vi "Actor-Run.vi"(8 "error in":errorcluster, 9 "Actor-Event-Registrations":T2, 10 "Actor-Events":T1, 11 "Actor in":refnum<class "Actor.lvclass">) -> (0 "error out":errorcluster, 3 "Actor out":refnum<class "Actor.lvclass">)   [LabVIEW 2018, in "Actor.lvlib" / "Actor.lvclass"]
uses:
  Actor.lvclass
  Event-Registrations.ctl
  Stop.ctl
  Events.ctl
  Launched.ctl
  Actor-Interface.lvclass
types:
  T1 = typedef "Actor.lvlib/Actor-Interface.lvclass/Events.ctl" = cluster{"Stop":refnum<user-event>, "Launched":refnum<user-event>}
  T2 = typedef "Actor.lvlib/Actor-Interface.lvclass/Event-Registrations.ctl" = cluster{"Stop":refnum<event-registration>}
  T3 = typedef "Actor.lvlib/Actor-Interface.lvclass/Launched.ctl" = cluster{"Actor":refnum<class "Actor.lvclass">}
  T4 = typedef "Actor.lvlib/Actor-Interface.lvclass/Stop.ctl" = enum16{"Normal", "Emergency"}
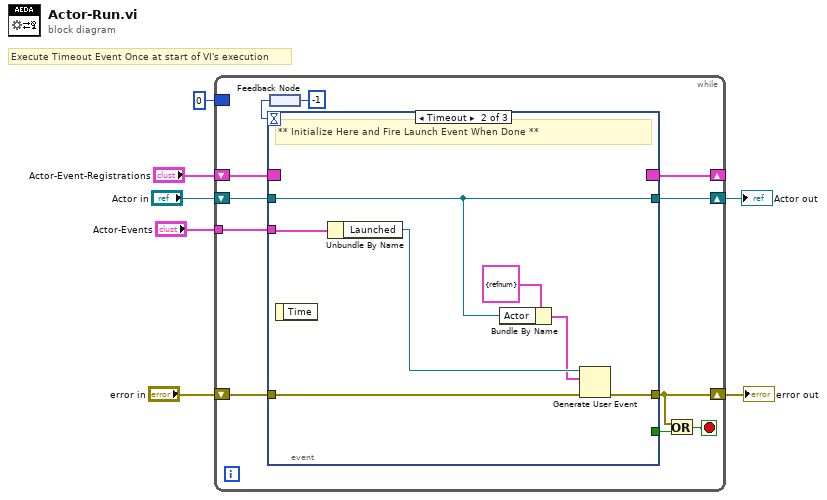
[diagram p0: block diagram]
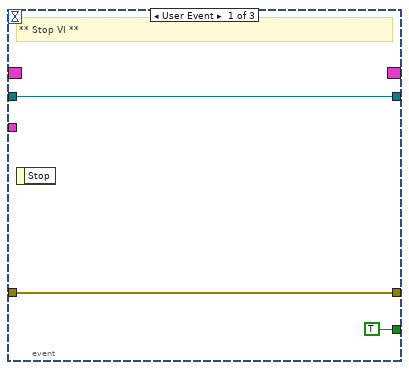
[diagram p2: hidden frame]
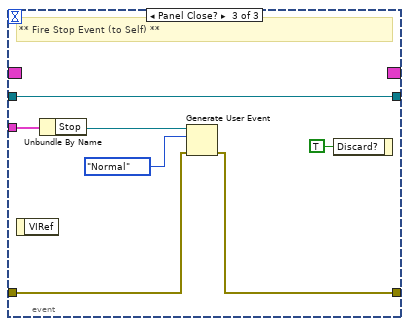
[diagram p3: hidden frame]
diagram:
  # "Execute Timeout Event Once at start of VI's execution"
  n1 = while {
    shift-right: [w13] -> w3
    shift-left: "Actor in" -> [w18]
    shift-right: [w12] -> w2
    shift-left: "error in" -> [w16]
    tunnel: "Actor-Events" -> [w15]
    shift-right: [w14] -> _
    shift-left: "Actor-Event-Registrations" -> [w17]
    border: 0 -> [_]
    stop <- w10 stop-if-true
    n2 = feedback-in #1(-1) -> ()
    n3 = feedback #1() -> (w8:i32)
    n4 = event shown="[1] Timeout" {
      selector: w17 -> [_ _ _]
      dyn-events: [_ _ _] -> w14
      timeout: w8 -> [_ _ _]
      tunnel: w18 -> [w21 w24 w34]
      tunnel: w16 -> [w20 w23 w31]
      tunnel: w15 -> [_ w28 w33]
      tunnel: [w21 w24 w34] -> w13
      tunnel: [w20 w22 w30] -> w12
      tunnel: [TRUE _ _] -> w11
      event User Event {
        # "** Stop VI **"
        n5 = event-data() -> ()  [unwired: 1 in, 1 out]
      }
      event Timeout {
        # "** Initialize Here and Fire Launch Event When Done **"
        n6 = event-data() -> ()  [unwired: 1 in, 1 out]
        n7 = Unbundle By Name(w28) -> ("Launched"=w27:refnum<user-event>)
        n8 = Bundle By Name(cluster=T3 {"Actor"=refnum} ("event data"), "Actor"=w24) -> (w25:T3)
        n9 = Generate User Event(user event=w27, event data cluster=w25, error in=w23) -> (error out=w22:errorcluster)  [unwired: 1 in, 1 out]
      }
      event Panel Close? {
        # "** Fire Stop Event (to Self) **"
        n10 = event-data() -> ()  [unwired: 1 in, 1 out]
        n11 = Unbundle By Name(w33) -> ("Stop"=w32:refnum<user-event>)
        n12 = Generate User Event(user event=w32, event data cluster=Stop."Normal" ("event data"), error in=w31) -> (error out=w30:errorcluster)  [unwired: 1 in, 1 out]
        n13 = event-data("Discard?"=TRUE) -> ()  [unwired: 1 in, 1 out]
      }
    }
    n14 = Or(x=w12, y=w11) -> (x .or. y?=w10:bool)
  }
  "error out" <- w2
  "Actor out" <- w3
